vi "From Pump Units.vi"(9 "Time Unit (0:second)":i32(ring)=1 items=["second"=1, "minute"=60, "hour"=3600], 10 "Volume Unit (1:mL)":i32(ring)=1000 items=["microliter"=1, "milliliter"=1000, "liter"=1000000], 11 "Value (0)":dbl) -> (2 "Acceleration":dbl, 3 "Flow rate":dbl)   [LabVIEW 2015, in "Global FIA milliGAT.lvlib"]
uses:
  Global FIA milliGAT.lvlib
panel:
  # "Note\nThis VI converts values returned by a pump (microliter, seconds) to the desired units."
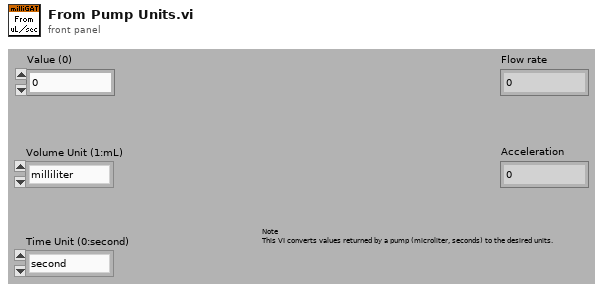
[diagram p1: front panel]
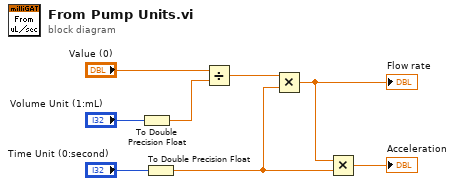
[diagram p0: block diagram]
diagram:
  n1 = To Double Precision Float(number="Volume Unit (1:mL)") -> (double precision float=w2:dbl)
  n2 = To Double Precision Float(number="Time Unit (0:second)") -> (double precision float=w1:dbl)
  n3 = Divide(x="Value (0)", y=w2) -> (x/y=w6:dbl)
  n4 = Multiply(x=w6, y=w1) -> (x*y=w5:dbl)
  "Flow rate" <- w5
  n5 = Multiply(x=w5, y=w1) -> (x*y=→"Acceleration":dbl)
